vi "fpga_ARC Compute Index Delay.vi"(2 "stepSize":u32, 3 "currSymbolIndex":i8, 4 "currFractional":u32) -> (0 "nextSymbolIndex":i8, 1 "nextFractionalDelay":u32)   [LabVIEW 2011, in "NI_EP_Resample_FPGA.lvlib"]
uses:
  <vilib>/rvi/FXPMathLib/basic elements/FxpAddSub/XNode/nifxpmath_AddSub.xnode
  <vilib>/addons/Electrical Power/PQ/Resampling/NI_EP_Resample_FPGA.lvlib
  <vilib>/rvi/FXPMathLib/sim/FxpSim.dll
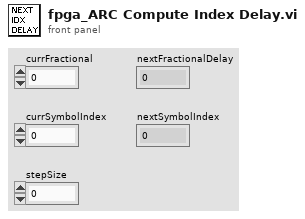
[diagram p1: front panel]
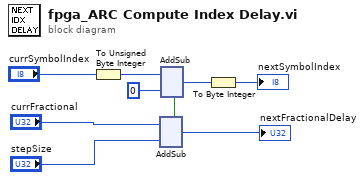
[diagram p0: block diagram]
diagram:
  n1 = To Unsigned Byte Integer(number="currSymbolIndex") -> (unsigned 8bit integer=w7:u8)
  n2 = xnode "AddSub"("x"="currFractional", "y"="stepSize") -> ("s"=→"nextFractionalDelay":u32, "carry-out"=w2:bool)
  n3 = xnode "AddSub"("x"=w7, "y"=u8 0, "carry-in"=w2) -> ("s"=w5:u8)  [unwired: 1 out]
  n4 = To Byte Integer(number=w5) -> (8bit integer=→"nextSymbolIndex":i8)
